vi "DAQmx Create Channel (AI-Resistance).vi"(0 "task in":refnum<k21>, 1 "maximum value":dbl=1000.0 format="%0.2f", 2 "minimum value":dbl=100.0 format="%0.2f", 3 "resistance configuration":i32(ring)=2 items=["2-Wire"=2, "3-Wire"=3, "4-Wire"=4], 5 "physical channels":tag, 7 "name to assign":string, 9 "units":i32(ring)=10384 items=["Ohms"=10384, "From Custom Scale"=10065], 10 "current excitation value":dbl=0.001 format="%0.5f", 11 "error in":errorcluster, 12 "custom scale name":tag, 13 "current excitation source":i32(ring)=10167 items=["Internal"=10200, "External"=10167, "None"=10230]) -> (4 "task out":refnum<k21>, 15 "error out":errorcluster)   [LabVIEW 2011]
doc: "Creates channel(s) to measure resistance."
uses:
  C:/Program Files/National Instruments/LabVIEW 2011/resource/objmgr/daqmx.rc
panel:
  # "input limits"
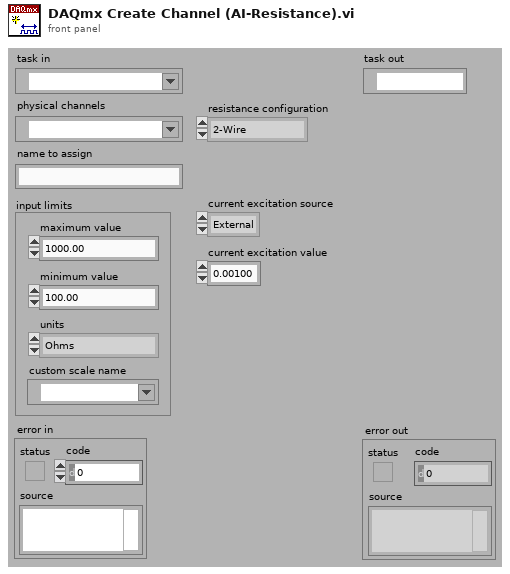
[diagram p1: front panel]
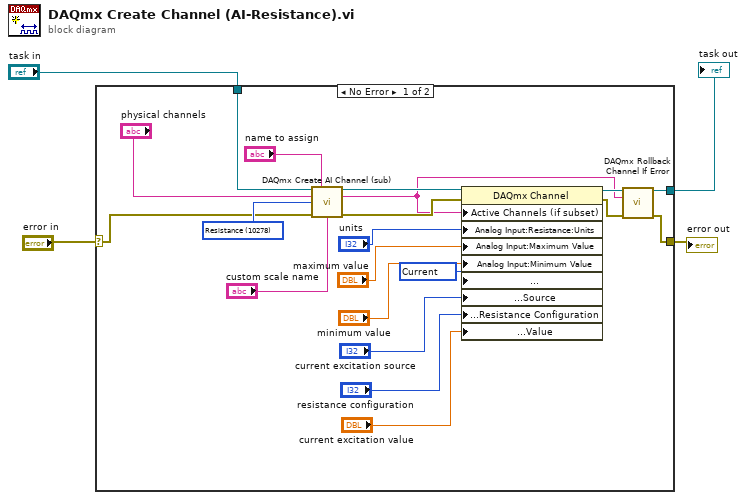
[diagram p0: block diagram]
diagram:
  n1 = case shown="No Error" "error in" {
    selector: "error in" -> [w12 w25]
    tunnel: [w6 w25] -> w4
    tunnel: "task in" -> [w24 w26]
    tunnel: [w7 w26] -> w1
    frame No Error {
      w10 = 10134 items=["Voltage"=10322, "Current"=10134] ("Analog Input:General Properties:Signal Conditioning:Excitation:Advanced:Voltage or Current")
      w14 = 10278 items=["Voltage"=10322, "Current"=10134, "More:Voltage:Custom with Excitation"=10323, "More:Current:Custom with Excitation"=10136, "Frequency"=10181, "Period"=10257, "Resistance"=10278, "Temperature:Thermocouple"=10303, "Temperature:Thermistor"=10302, "Temperature:RTD"=10301, "Temperature:Built-in Sensor"=10311, "Strain Gage"=10300] ("measurement type")
      n2 = call "DAQmx Create AI Channel (sub).vi"("task in"=w24, "virtual channel name"="name to assign", "physical channel name"="physical channels", "measurement type"=w14, "error in"=w12, "custom scale"="custom scale name") -> ("task out"=w11:refnum<k21>, "channel names"=w5:string, "error out"=w22:errorcluster)  [unwired: 7 out]
      n3 = property class="DAQmx Channel"(reference=w11, error in=w22, "Active Channels (if subset)"=w5, "Analog Input:Resistance:Units"="units", "Analog Input:Maximum Value"="maximum value", "Analog Input:Minimum Value"="minimum value", "Analog Input:General Properties:Signal Conditioning:Excitation:Advanced:Voltage or Current"=w10, "Analog Input:General Properties:Signal Conditioning:Excitation:Source"="current excitation source", "Analog Input:General Properties:Signal Conditioning:Resistance Configuration"="resistance configuration", "Analog Input:General Properties:Signal Conditioning:Excitation:Value"="current excitation value") -> (reference out=w9:refnum<k21>, error out=w8:errorcluster)
      n4 = call "DAQmx Rollback Channel If Error.vi"("task in"=w9, "channel names"=w5, "error in"=w8) -> ("task out"=w7:refnum<k21>, "error out"=w6:errorcluster)  [unwired: 11 out]
    }
    frame Error {
    }
  }
  "error out" <- w4
  "task out" <- w1
